vi "Add UEGO Card From Table.vi"(8 "error in (no error)":errorcluster, 10 "Card Position":T1={"Rack #"=0, "Slot #"=1} {"Slot #" max=15}, 11 "Node Ptr":u64 format="%.0x") -> (0 "error out":errorcluster)   [LabVIEW 2014, in "SLSC configuration System Explorer.lvlib"]
uses:
  SLSC configuration System Explorer.lvlib
  Type Defs/Card Position.ctl
  Shared/SPI Utility/Slot #.ctl
  Shared/Constants.vi
  Shared/SLSC configuration Shared.lvlib
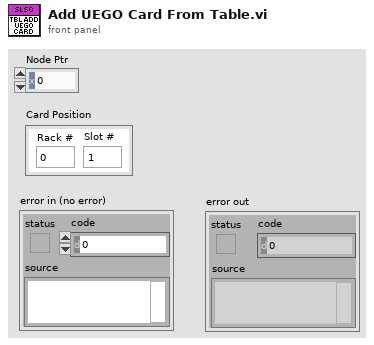
[diagram p1: front panel]
types:
  T1 = typedef "SLSC configuration Shared.lvlib/Card Position.ctl" = cluster{"Rack #":u8, "Slot #":T2}
  T2 = typedef "SLSC configuration Shared.lvlib/Slot #.ctl" = u8
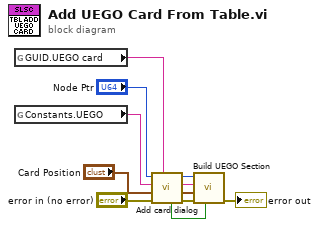
[diagram p0: block diagram]
diagram:
  n1 = global read "Constants.vi" "GUID.UEGO card"() -> (w1:string)
  n2 = global read "Constants.vi" "Constants.UEGO"() -> (w5:string)
  n3 = call "Add card dialog.vi"("Card GUID"=w1, "error in (no error)"="error in (no error)", "Card Position"="Card Position", "Card Type in"=w5, "Node Ptr"="Node Ptr") -> ("error out"=w9:errorcluster, "Card Position out"=w6:T1, "Name out"=w8:string, "Node Ptr out"=w7:u64, "Cancelled?"=w3:bool)  [unwired: 2 in]
  n4 = call "Build UEGO Section.vi"("Cancelled?"=w3, "error in (no error)"=w9, "Card Position in"=w6, "Name in"=w8, "Node Ptr in"=w7) -> ("error out"=→"error out":errorcluster)  [unwired: 6 in]
